vi "Timer.vi"(0 "Module Data In":T2, 5 "Mode":T1, 7 "Update Target?":bool, 9 "Time Target":dbl, 11 "error in (no error)":errorcluster) -> (4 "Module Data Out":T2, 6 "Reached?":bool, 8 "Elapsed Time":dbl, 15 "error out":errorcluster)   [LabVIEW 2017, in "Error Handler - Logger.lvlib"]
doc: "Every time this Vi is called in read mode, it will increment the time elasped since its last call.\nThe time counter can also be paused and resumed."
uses:
  Error Handler - Logger.lvlib
  Controls/Module - Data.ctl
  Modules.ctl
  Controls/Module - States.ctl
  Controls/Timing - Data.ctl
  Controls/Process - Element.ctl
  Controls/Process.ctl
  Controls/Process - Status.ctl
  Controls/Current Error Details.ctl
  Controls/Error Types.ctl
  Controls/Timing - Mode.ctl
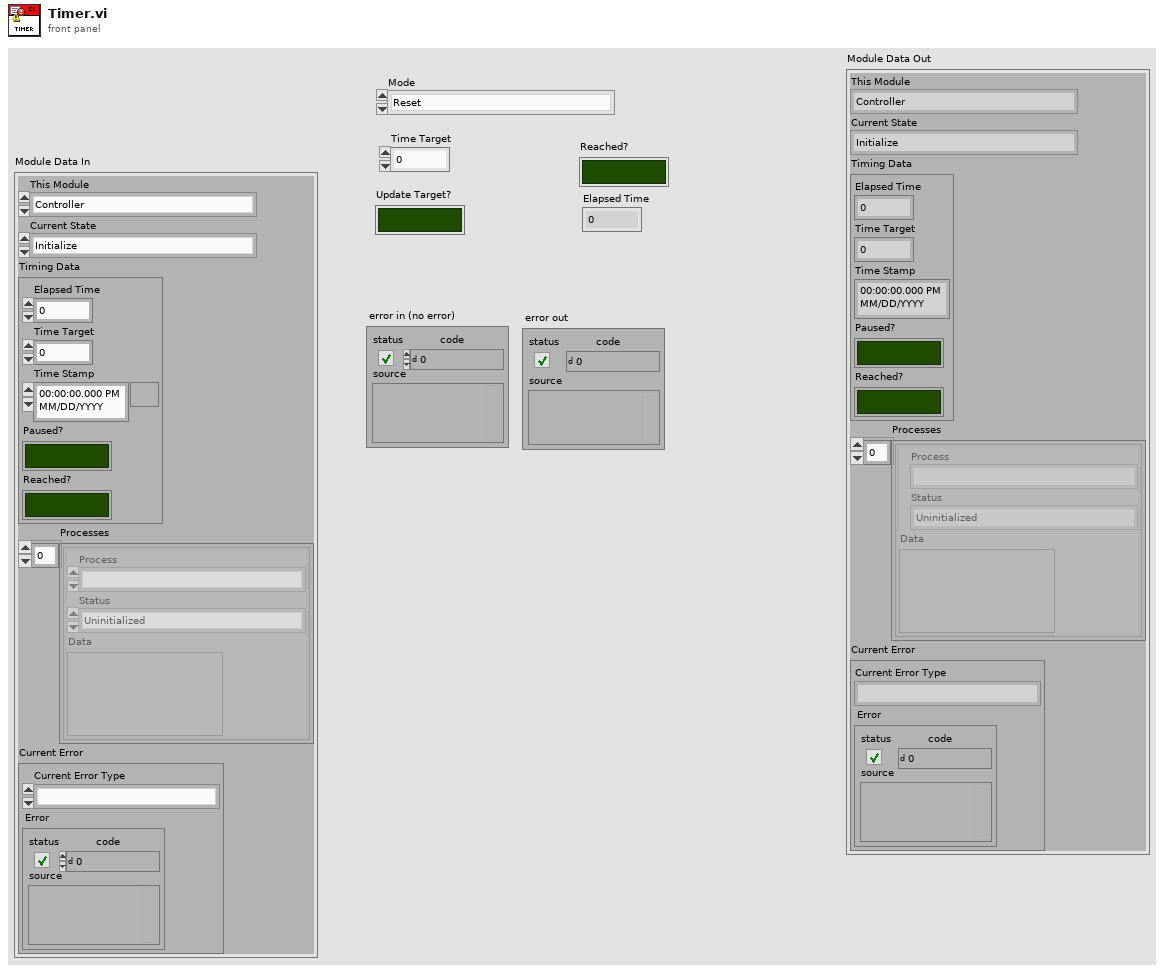
[diagram p1: front panel]
types:
  T1 = typedef "Error Handler - Logger.lvlib/Timing - Mode.ctl" = enum16{"Reset", "Read", "Pause", "Resume"}
  T2 = typedef "Error Handler - Logger.lvlib/Module - Data.ctl" = cluster{"This Module":T3, "Current State":T4, "Timing Data":T5, "Processes":T6[], "Current Error":T9}
  T3 = typedef "Error Handler - Logger.lvlib/Modules.ctl" = enum16{"Controller", "Error Handler - Logger"}
  T4 = typedef "Error Handler - Logger.lvlib/Module - States.ctl" = enum16{"Initialize", "Event ", "Send data", "FP Element: Update", "FP Element: Disable/Enable", "Timer: Setup", "Terminate", "--------Template----------", "Process Error", "Log ", "Log Error"}
  T5 = typedef "Error Handler - Logger.lvlib/Timing - Data.ctl" = cluster{"Elapsed Time":dbl, "Time Target":dbl, "Time Stamp":timestamp, "Paused?":bool, "Reached?":bool}
  T6 = typedef "Error Handler - Logger.lvlib/Process - Element.ctl" = cluster{"Process":T7, "Status":T8, "Data":variant}
  T7 = typedef "Error Handler - Logger.lvlib/Process.ctl" = enum16{""}
  T8 = typedef "Error Handler - Logger.lvlib/Process - Status.ctl" = enum16{"Uninitialized", "Busy"}
  T9 = typedef "Error Handler - Logger.lvlib/Current Error Details.ctl" = cluster{"Current Error Type":T10, "Error":errorcluster}
  T10 = typedef "Error Handler - Logger.lvlib/Error Types.ctl" = enum16{""}
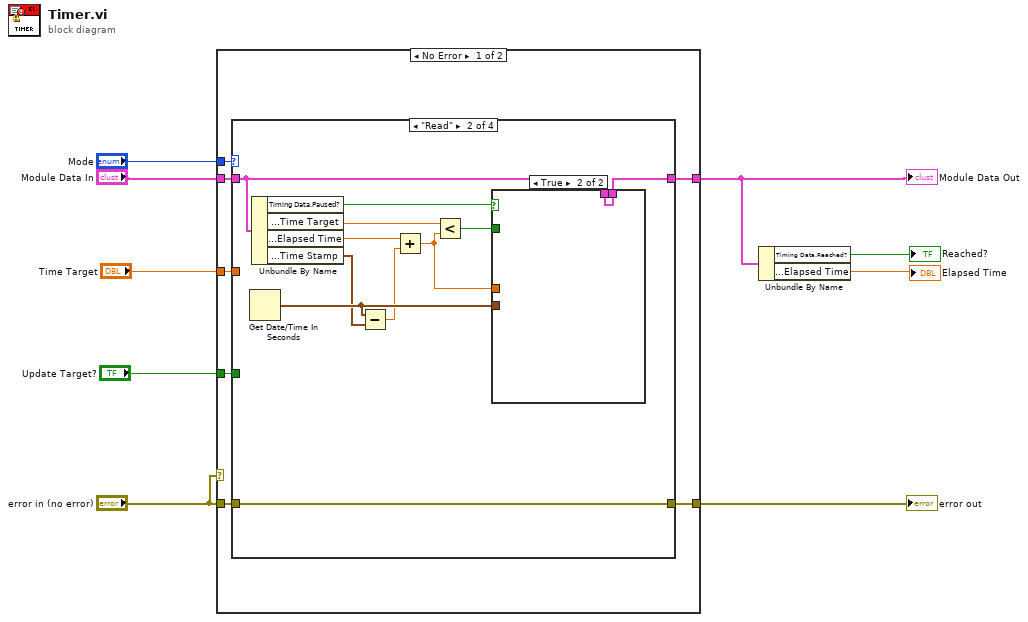
[diagram p0: block diagram]
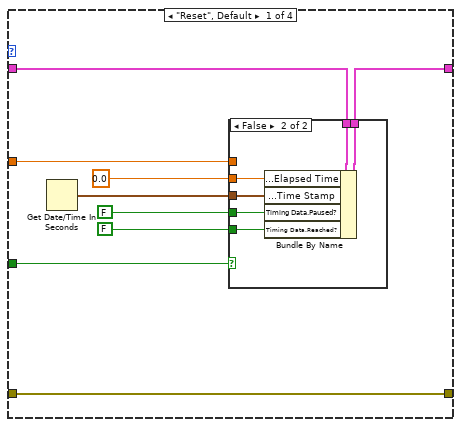
[diagram p2: hidden frame]
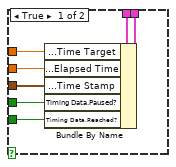
[diagram p3: hidden frame]
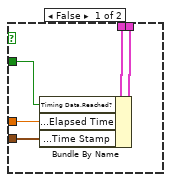
[diagram p4: hidden frame]
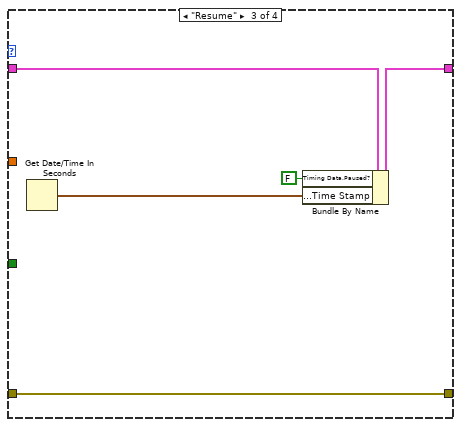
[diagram p5: hidden frame]
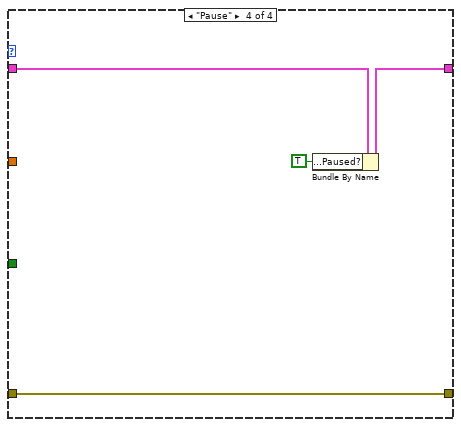
[diagram p6: hidden frame]
diagram:
  n1 = case shown="No Error" "error in (no error)" {
    tunnel: [w16 w66] -> w3
    tunnel: "Module Data In" -> [w15 w66]
    tunnel: [w14 w65] -> w8
    tunnel: "error in (no error)" -> [w13 w65]
    tunnel: "Mode" -> [w12 _]
    tunnel: "Update Target?" -> [w11 _]
    tunnel: "Time Target" -> [w10 _]
    frame No Error {
      n2 = case shown="\"Read\"" w12 {
        tunnel: [w23 w48 w59 w63] -> w16
        tunnel: w15 -> [w24 w47 w58 w62]
        tunnel: [w25 w49 w60 w64] -> w14
        tunnel: w13 -> [w25 w49 w60 w64]
        tunnel: w11 -> [w19 _ _ _]
        tunnel: w10 -> [w17 _ _ _]
        frame "Reset", Default {
          n3 = Get Date/Time In Seconds() -> (seconds since 1Jan1904=w20:timestamp)
          n4 = case shown="False" w19 {
            tunnel: w24 -> [w32 w38]
            tunnel: [w31 w37] -> w23
            tunnel: FALSE ("Timing Data.Paused?") -> [w30 w36]
            tunnel: FALSE ("Timing Data.Reached?") -> [w29 w35]
            tunnel: w20 -> [w28 w34]
            tunnel: 0.0 ("Timing Data.Elapsed Time") -> [w27 w33]
            tunnel: w17 -> [w26 _]
            frame True {
              n5 = Bundle By Name(cluster=w32, "Timing Data.Time Target"=w26, "Timing Data.Elapsed Time"=w27, "Timing Data.Time Stamp"=w28, "Timing Data.Paused?"=w30, "Timing Data.Reached?"=w29) -> (w31:T2)
            }
            frame False {
              n6 = Bundle By Name(cluster=w38, "Timing Data.Elapsed Time"=w33, "Timing Data.Time Stamp"=w34, "Timing Data.Paused?"=w36, "Timing Data.Reached?"=w35) -> (w37:T2)
            }
          }
        }
        frame "Read" {
          n7 = Get Date/Time In Seconds() -> (seconds since 1Jan1904=w46:timestamp)
          n8 = Unbundle By Name(w47) -> ("Timing Data.Paused?"=w39:bool, "Timing Data.Time Target"=w42:dbl, "Timing Data.Elapsed Time"=w44:dbl, "Timing Data.Time Stamp"=w45:timestamp)
          n9 = Subtract(x=w46, y=w45) -> (x-y=w43:dbl)
          n10 = Add(x=w44, y=w43) -> (x+y=w41:dbl)
          n11 = Less?(x=w42, y=w41) -> (x < y?=w40:bool)
          n12 = case shown="True" w39 {
            tunnel: [w54 w55] -> w48
            tunnel: w47 -> [w53 w55]
            tunnel: w46 -> [w52 _]
            tunnel: w41 -> [w51 _]
            tunnel: w40 -> [w50 _]
            frame False {
              n13 = Bundle By Name(cluster=w53, "Timing Data.Reached?"=w50, "Timing Data.Elapsed Time"=w51, "Timing Data.Time Stamp"=w52) -> (w54:T2)
            }
            frame True {
            }
          }
        }
        frame "Resume" {
          n14 = Get Date/Time In Seconds() -> (seconds since 1Jan1904=w57:timestamp)
          n15 = Bundle By Name(cluster=w58, "Timing Data.Paused?"=FALSE, "Timing Data.Time Stamp"=w57) -> (w59:T2)
        }
        frame "Pause" {
          n16 = Bundle By Name(cluster=w62, "Timing Data.Paused?"=TRUE) -> (w63:T2)
        }
      }
    }
    frame Error {
    }
  }
  "error out" <- w8
  "Module Data Out" <- w3
  n17 = Unbundle By Name(w3) -> ("Timing Data.Reached?"=→"Reached?":bool, "Timing Data.Elapsed Time"=→"Elapsed Time":dbl)
